vi "siave_serial.vi"(8 "error in (no error)":errorcluster, 9 "velocidade":dbl, 10 "k":dbl, 11 "VISA resource name":refnum<visa-resource-name>) -> (0 "error out":errorcluster, 2 "ok":bool, 3 "VISA resource name out":refnum<visa-resource-name>, 4 "Umidade":dbl, 6 "Temp":dbl)   [LabVIEW 2010]
doc: "Envia comando para SIAVE Velocidade e k, recebe confirmação e dados Temperatura e Umidade, se disponíveis."
uses:
  <vilib>/Instr/_visa.llb/VISA Configure Serial Port (Instr).vi
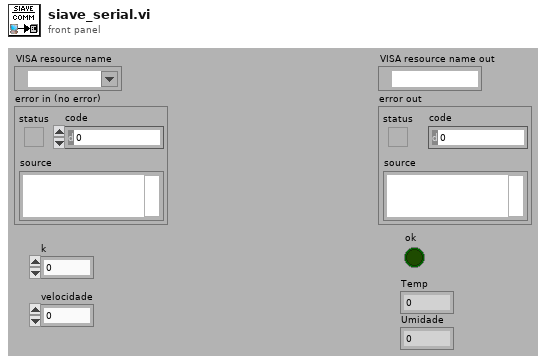
[diagram p1: front panel]
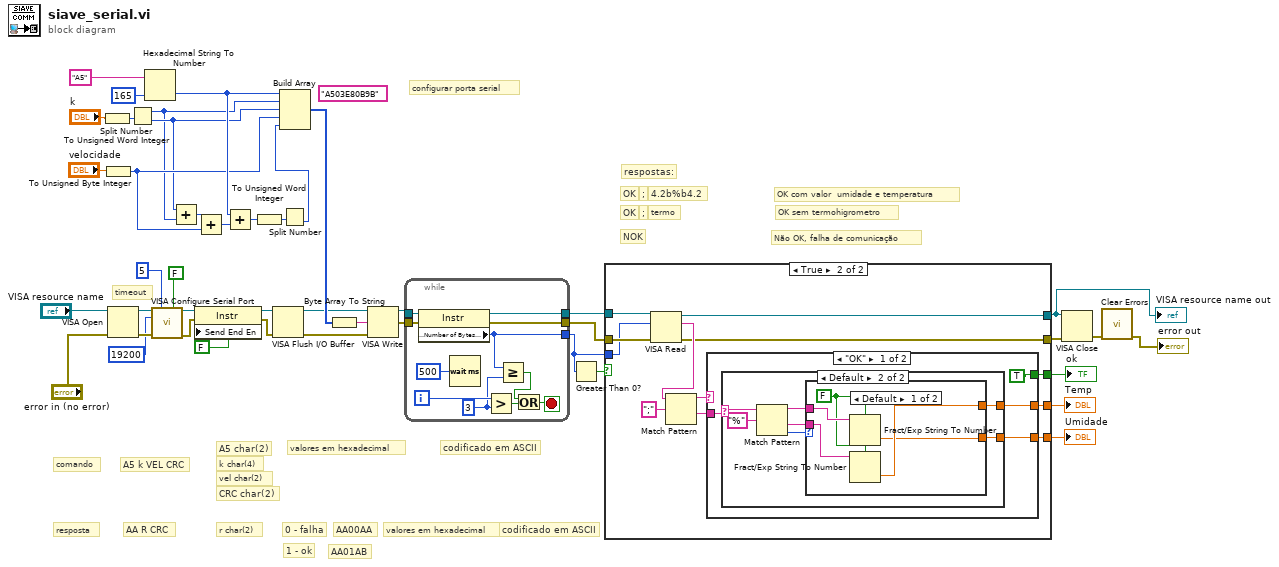
[diagram p0: block diagram]
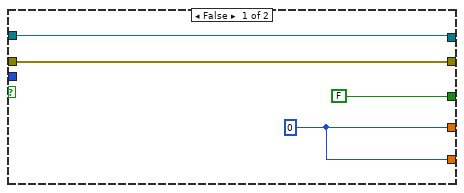
[diagram p2: hidden frame]
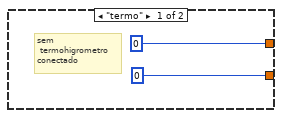
[diagram p3: hidden frame]
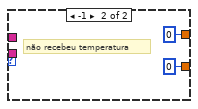
[diagram p4: hidden frame]
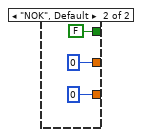
[diagram p5: hidden frame]
diagram:
  (unwired) "A503E80B9B"
  # "configurar porta serial"
  # "timeout"
  # ";"
  # ";"
  # "termo"
  # "respostas:"
  # "Não OK, falha de comunicação"
  # "OK sem termohigrometro"
  # "OK com valor  umidade e temperatura"
  # "4.2b%b4.2"
  # "NOK"
  # "OK"
  # "OK"
  # "AA00AA"
  # "AA01AB"
  # "codificado em ASCII"
  # "codificado em ASCII"
  # "valores em hexadecimal"
  # "valores em hexadecimal"
  # "A5 char(2)"
  # "1 - ok"
  # "0 - falha"
  # "r char(2)"
  # "CRC char(2)"
  # "vel char(2)"
  # "k char(4)"
  # "AA R CRC"
  # "A5 k VEL CRC"
  # "resposta"
  # "comando"
  n1 = To Unsigned Word Integer(number="k") -> (unsigned 16bit integer=w34:u16)
  n2 = To Unsigned Byte Integer(number="velocidade") -> (unsigned 8bit integer=w29:u8)
  n3 = VISA Open(error in (no error)="error in (no error)", VISA resource name="VISA resource name") -> (VISA resource name=w14:refnum<visa-resource-name>, error out=w15:errorcluster)  [unwired: 3 in]
  n4 = Split Number(x=w34) -> (hi(x)=w27:u8, lo(x)=w28:u8)
  n5 = Hexadecimal String To Number(string="A5", default (0uL)=u8 165 ("default (0 U32)")) -> (number=w32:u8)  [unwired: 1 in, 1 out]
  n6 = call-poly "VISA Configure Serial Port"("VISA resource name"=w14, "timeout (10sec)"=u32 5, "Enable Termination\nChar (T)"=FALSE ("Message Based Settings:Send End Enable"), "baud rate (9600)"=u32 19200, "error in (no error)"=w15) -> ("VISA resource name out"=w13:refnum<visa-resource-name>, "error out"=w12:errorcluster)  [unwired: 9 in]
  n7 = Add(x=w28, y=w27) -> (x+y=w30:u8)
  n8 = property class="Instr"(reference=w13, error in=w12, "Send End En"=FALSE ("Message Based Settings:Send End Enable")) -> (reference out=w8:refnum<visa-resource-name>, error out=w7:errorcluster)
  n9 = Add(x=w30, y=w29) -> (x+y=w43:u8)
  n10 = Add(x=w32, y=w43) -> (x+y=w37:u8)
  n11 = To Unsigned Word Integer(number=w37) -> (unsigned 16bit integer=w41:u16)
  n12 = VISA Flush I/O Buffer(VISA resource name=w8, error in (no error)=w7) -> (VISA resource name out=w22:refnum<visa-resource-name>, error out=w21:errorcluster)  [unwired: 1 in]
  n13 = Split Number(x=w41) -> (lo(x)=w31:u8)  [unwired: 1 out]
  n14 = Build Array(w32, w27, w28, w29, w31) -> (w25:u8[])
  n15 = Byte Array To String(unsigned byte array=w25) -> (string=w26:string)
  n16 = VISA Write(VISA resource name=w22, write buffer=w26, error in (no error)=w21) -> (VISA resource name out=w18:refnum<visa-resource-name>, error out=w17:errorcluster)  [unwired: 1 out]
  n17 = while {
    tunnel: [w54] -> w40
    tunnel: [w53] -> w39
    tunnel: [w48] -> w24
    tunnel: w18 -> [w52]
    tunnel: w17 -> [w51]
    i -> [w49]
    stop <- w44 stop-if-true
    w47 = 3 ("y")
    n18 = property class="Instr"(reference=w52, error in=w51) -> (reference out=w54:refnum<visa-resource-name>, error out=w53:errorcluster, "Serial Settings:Number of Bytes at Serial Port"=w48:u32)
    n19 = Wait (ms)(milliseconds to wait=u32 500) -> ()  [unwired: 1 out]
    n20 = Greater?(x=w49, y=w47) -> (0:w46:bool)
    n21 = Greater Or Equal?(x=w48, y=w47) -> (x >= y?=w45:bool)
    n22 = Or(x=w45, y=w46) -> (x .or. y?=w44:bool)
  }
  n23 = Greater Than 0?(x=w24) -> (x > 0?=w38:bool)
  n24 = case shown="True" w38 {
    tunnel: [w57 w59] -> w3
    tunnel: [w58 w70] -> w1
    tunnel: w40 -> [w58 w69]
    tunnel: w39 -> [w57 w68]
    tunnel: w24 -> [_ w67]
    tunnel: [FALSE w63] -> w23
    tunnel: [w55 w61] -> w20
    tunnel: [w55 w60] -> w19
    frame False {
      w55 = 0
    }
    frame True {
      n25 = VISA Read(VISA resource name=w69, byte count=w67, error in (no error)=w68) -> (VISA resource name out=w70:refnum<visa-resource-name>, read buffer=w65:string, error out=w59:errorcluster)  [unwired: 1 out]
      n26 = Match Pattern(string=w65, regular expression=";") -> (before substring=w64:string, after substring=w62:string)  [unwired: 1 in, 2 out]
      n27 = case shown="\"OK\"" w64 {
        tunnel: [TRUE FALSE] -> w63
        tunnel: w62 -> [w74 _]
        tunnel: [w73 0] -> w61
        tunnel: [w72 0] -> w60
        frame "OK" {
          n28 = case shown="Default" w74 {
            selector: w74 -> [_ w83]
            tunnel: [0 w81] -> w73
            tunnel: [0 w80] -> w72
            frame "termo" {
              # "sem\n termohigrometro\nconectado"
            }
            frame Default {
              n29 = Match Pattern(string=w83, regular expression="%") -> (before substring=w78:string, after substring=w77:string, offset past match=w79:i32)  [unwired: 1 in, 1 out]
              n30 = case shown="Default" w79 {
                tunnel: [w85 0] -> w81
                tunnel: [w84 0] -> w80
                tunnel: w78 -> [w88 _]
                tunnel: w77 -> [w87 _]
                frame Default {
                  w86 = FALSE ("use system decimal point (T)")
                  n31 = Fract/Exp String To Number(use system decimal point (T)=w86, string=w88) -> (number=w84:dbl)  [unwired: 2 in, 1 out]
                  n32 = Fract/Exp String To Number(use system decimal point (T)=w86, string=w87) -> (number=w85:dbl)  [unwired: 2 in, 1 out]
                }
                frame -1 {
                  # "não recebeu temperatura"
                }
              }
            }
          }
        }
        frame "NOK", Default {
        }
      }
    }
  }
  "VISA resource name out" <- w1
  "ok" <- w23
  "Temp" <- w20
  "Umidade" <- w19
  n33 = VISA Close(VISA resource name=w1, error in (no error)=w3) -> (error out=w4:errorcluster)
  n34 = call <vilib>:"Clear Errors.vi"("error in (no error)"=w4) -> ("error out"=→"error out":errorcluster)  [unwired: 6 in]
